vi "LM Lorentzian-Gaussian and gradient.vi"(3 "output control":T1, 4 "data":variant, 5 "X":dbl[](array[numeric]), 6 "a":dbl[](array[numeric])) -> (0 "error out":errorcluster, 1 "f'(X,a)":dbl[][](array[numeric]), 2 "f(X,a)":dbl[](array[numeric]))   [LabVIEW 2021, in "Fits.lvlib"]
doc: "This template is the starting point for creating a model function to be passed to the Nonlinear Curve Fit.vi."
uses:
  <vilib>/gmath/NumericalOptimization/LM_output select.ctl
  Fits.lvlib
  <vilib>/gmath/NI_Gmath.lvlib
panel:
  # "Parameters:\n\namplitude: A\ncenter: t_0\nFWHM-: w-\nSDV+: s+"
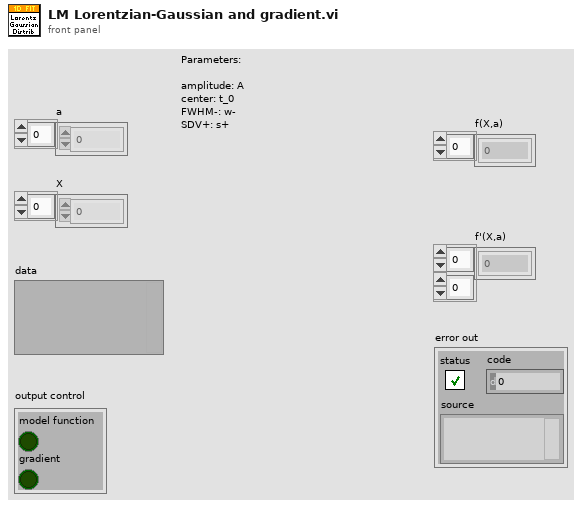
[diagram p1: front panel]
types:
  T1 = typedef "NI_Gmath.lvlib/LM_output select.ctl" = cluster{"model function":bool, "gradient":bool}
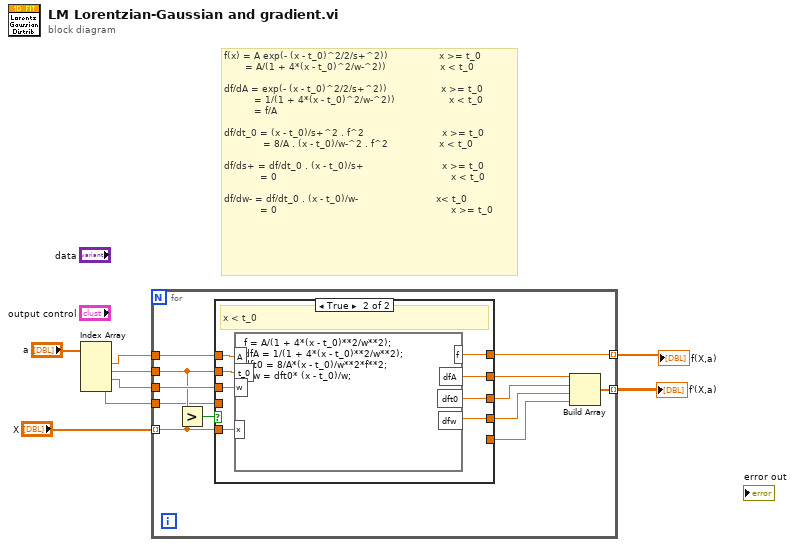
[diagram p0: block diagram]
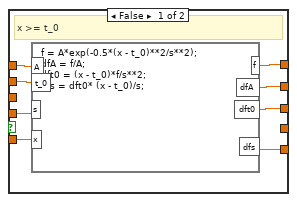
[diagram p2: hidden frame]
diagram:
  # "f(x) = A exp(- (x - t_0)^2/2/s+^2))                 x >= t_0\n       = A/(1 + 4*(x - t_0)^2/w-^2))                  x < t_0\n\ndf/dA = exp(- (x - t_0)^2/2/s+^2))                  x >= t_0\n          = 1/(1 + 4*(x - t_0)^2/w-^2))                  x < t_0\n          = f/A\n\ndf/dt_0 = (x - t_0)/s+^2 . f^2                          x >= t_0\n             = 8/A . (x - t_0)/w-^2 . f^2                 x < t_0\n\ndf/ds+ = df/dt_0 . (x - t_0)/s+                          x >= t_0\n            = 0                                                          x < t_0\n\ndf/dw- = df/dt_0 . (x - t_0)/w-                          x< t_0\n            = 0                                                          x >= t_0"
  n1 = Index Array(array="a") -> (element #1=w7:dbl, element #2=w6:dbl, element #3=w5:dbl, element #4=w4:dbl)  [unwired: 4 in]
  n2 = for {
    tunnel: w7 -> [w20]
    tunnel: w6 -> [w18]
    tunnel: w5 -> [w19]
    tunnel: w4 -> [w11]
    tunnel: "X" -> [w17] mode=indexing
    tunnel: [w15] -> w2 mode=indexing
    tunnel: [w13] -> w1 mode=indexing
    n3 = Greater?(x=w18, y=w17) -> (0:w12:bool)
    n4 = case shown="True" w12 {
      tunnel: w20 -> [w28 w36]
      tunnel: w19 -> [_ w30]
      tunnel: w18 -> [w27 w35]
      tunnel: w17 -> [w26 w34]
      tunnel: [w24 w33] -> w16
      tunnel: [w25 w32] -> w15
      tunnel: [w23 w31] -> w14
      tunnel: w11 -> [w22 _]
      tunnel: [_ w29] -> w10
      tunnel: [w21 _] -> w9
      frame False {
        # "x >= t_0"
        n5 = formula code="f = A*exp(-0.5*(x - t_0)**2/s**2);\ndfA = f/A;\ndft0 = (x - t_0)*f/s**2;\ndfs = dft0* (x - t_0)/s;"("A"=w28, "t_0"=w27, "s"=w22, "x"=w26) -> ("f"=w25:dbl, "dfA"=w24:dbl, "dft0"=w23:dbl, "dfs"=w21:dbl)
      }
      frame True {
        # "x < t_0"
        n6 = formula code="f = A/(1 + 4*(x - t_0)**2/w**2);\ndfA = 1/(1 + 4*(x - t_0)**2/w**2);\ndft0 = 8/A*(x - t_0)/w**2*f**2;\ndfw = dft0* (x - t_0)/w;"("A"=w36, "t_0"=w35, "w"=w30, "x"=w34) -> ("f"=w32:dbl, "dfA"=w33:dbl, "dft0"=w31:dbl, "dfw"=w29:dbl)
      }
    }
    n7 = Build Array(w16, w14, w10, w9) -> (w13:dbl[])
  }
  "f(X,a)" <- w2
  "f'(X,a)" <- w1
